vi "lv_to_cstr.vi"(8 "error in (no error)":errorcluster, 11 "labview string":string) -> (0 "error out":errorcluster, 3 "C string":u64)   [LabVIEW 2023, in "uhd.lvlib"]
uses:
  <userlib>/uhd/uhd.lvlib
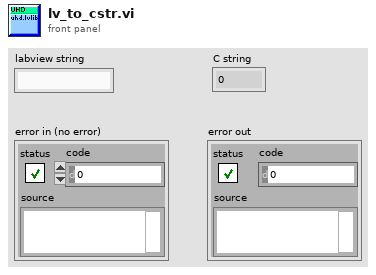
[diagram p1: front panel]
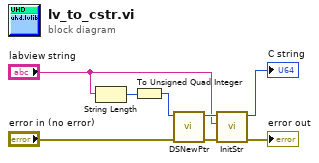
[diagram p0: block diagram]
diagram:
  n1 = String Length(string="labview string") -> (length=w2:i32)
  n2 = To Unsigned Quad Integer(1:w2) -> (0:w1:u64)
  n3 = call <vilib>:"DSNewPtr.vi"("error in (no error)"="error in (no error)", "Size"=w1) -> ("error out"=w4:errorcluster, "Pointer"=w8:u64)  [unwired: 8 in]
  n4 = call <vilib>:"InitStr.vi"("error in (no error)"=w4, "ConstCStr"="labview string", "Pointer"=w8) -> ("error out"=→"error out":errorcluster, "CStrP"=→"C string":u64)  [unwired: 7 in]
